vi "cmd check.vi"(8 "error in (no error)":errorcluster, 11 "motor in":refnum<class "AISAS motor.lvclass">) -> (0 "error out":errorcluster, 1 "Motor Ok?":bool, 3 "motor out":refnum<class "AISAS motor.lvclass">)   [LabVIEW 2014, in "AISAS motor.lvclass"]
uses:
  AISAS motor.lvclass
  Controls/motor.ctl
  AISAS motor.lvclass/AISAS motor.ctl
panel:
  out "Motor":T1
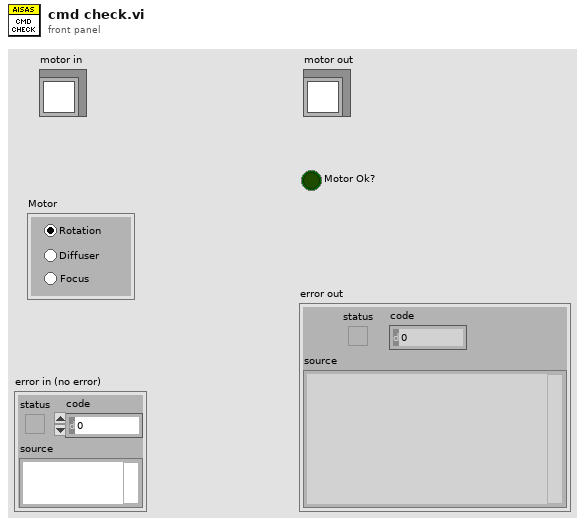
[diagram p1: front panel]
types:
  T1 = typedef "motor.ctl" = enum32{"Rotation", "Diffuser ", "Focus"}
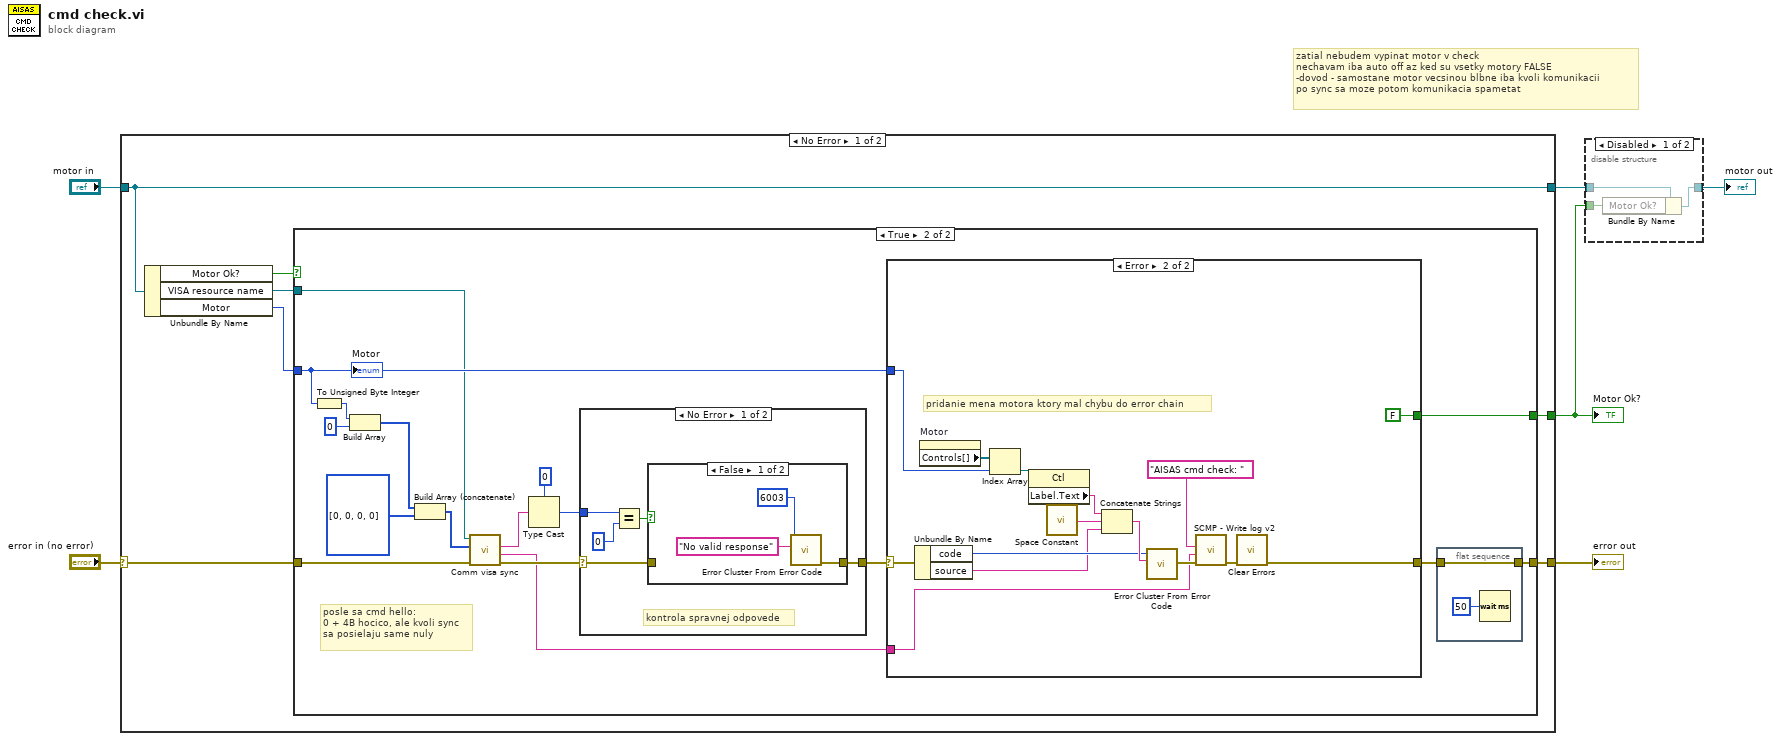
[diagram p0: block diagram]
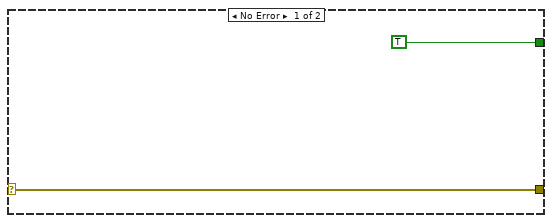
[diagram p4: hidden frame]
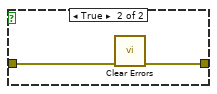
[diagram p5: hidden frame]
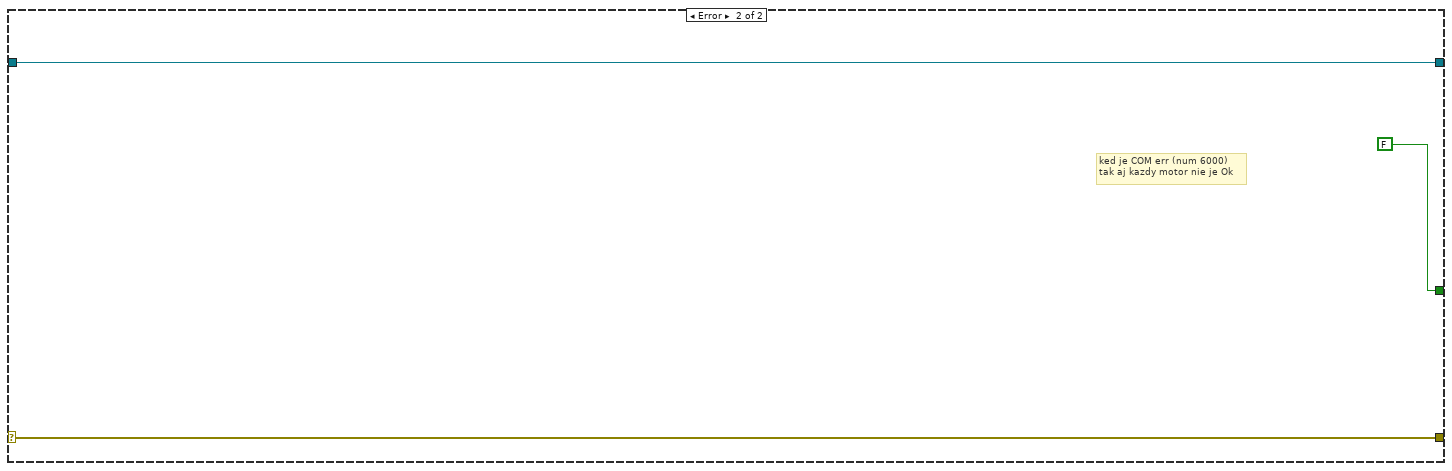
[diagram p7: hidden frame]
diagram:
  # "zatial nebudem vypinat motor v check\nnechavam iba auto off az ked su vsetky motory FALSE\n-dovod - samostane motor vecsinou blbne iba kvoli komunikacii\npo sync sa moze potom komunikacia spametat"
  n1 = case shown="No Error" "error in (no error)" {
    selector: "error in (no error)" -> [w11 w65]
    tunnel: [w13 w65] -> w5
    tunnel: "motor in" -> [w9 w64]
    tunnel: [w10 FALSE ("Motor Ok")] -> w3
    tunnel: [w9 w64] -> w2
    frame No Error {
      n2 = Unbundle By Name(w9) -> ("Motor Ok?"=w7:bool, "VISA resource name"=w8:refnum<visa-resource-name>, "Motor"=w12:T1)
      n3 = case shown="True" w7 {
        selector: w7 -> [w14 _]
        tunnel: [w14 w31] -> w10
        tunnel: [w15 w22] -> w13
        tunnel: w12 -> [_ w27]
        tunnel: w11 -> [w15 w25]
        tunnel: w8 -> [_ w16]
        frame False {
        }
        frame True {
          # "posle sa cmd hello:\n0 + 4B hocico, ale kvoli sync\nsa posielaju same nuly"
          n4 = To Unsigned Byte Integer(number=w27) -> (unsigned 8bit integer=w20:u8)
          n5 = Build Array(w20, u8 0) -> (w18:u8[])
          n6 = Build Array (concatenate)(w18, u8[] [0, 0, 0, 0]) -> (w17:u8[])
          n7 = call "Comm visa sync.vi"("error in (no error)"=w25, "Command"=w17, "VISA in"=w16) -> ("error out"=w30:errorcluster, "sync info"=w21:string, "Response"=w26:string)  [unwired: 5 in, 1 out]
          n8 = Type Cast(type=u8 0, x=w26) -> (*(type *) &x=w28:u8)
          n9 = case shown="No Error" w30 {
            selector: w30 -> [w56 w62]
            tunnel: [w54 w62] -> w32
            tunnel: w28 -> [w52 _]
            frame No Error {
              # "kontrola spravnej odpovede"
              n10 = Equal?(x=w52, y=u8 0) -> (x = y?=w55:bool)
              n11 = case shown="False" w55 {
                tunnel: w56 -> [_ w61]
                tunnel: [w57 w60] -> w54
                frame False {
                  n12 = call <vilib>:"Error Cluster From Error Code.vi"("error message (\"\")"="No valid response" ("error message (\"\")"), "error code (0)"=6003) -> ("error out"=w57:errorcluster)  [unwired: 7 in]
                }
                frame True {
                  n13 = call <vilib>:"Clear Errors.vi"("error in (no error)"=w61) -> ("error out"=w60:errorcluster)  [unwired: 5 in, 1 out]
                }
              }
            }
            frame Error {
            }
          }
          n14 = case shown="Error" w32 {
            selector: w32 -> [w35 w47]
            tunnel: [TRUE ("Motor Ok") FALSE ("Motor Ok")] -> w31
            tunnel: w27 -> [_ w48]
            tunnel: [w35 w37] -> w23
            tunnel: w21 -> [_ w38]
            frame No Error {
            }
            frame Error {
              # "pridanie mena motora ktory mal chybu do error chain"
              n15 = Unbundle By Name(w47) -> ("code"=w45:i32, "source"=w44:string)
              n16 = property on="Motor" class="RadioBtnsControl (strict)"() -> ("Controls[]"=w50:refnum<vi>[])  [unwired: 2 in, 2 out]
              n17 = Index Array(array=w50, index=w48) -> (element=w49:refnum<vi>)
              n18 = property class="Ctl"(reference=w49) -> ("Label.Text"=w43:string)  [unwired: 1 in, 2 out]
              n19 = call <vilib>:"Space Constant.vi"() -> ("String"=w42:string)
              n20 = Concatenate Strings(w43, w42, w44) -> (w46:string)
              n21 = call <vilib>:"Error Cluster From Error Code.vi"("error message (\"\")"=w46, "error code (0)"=w45) -> ("error out"=w41:errorcluster)  [unwired: 7 in]
              n22 = call "SCMP - Write log v2.vi"("Error to log"=w41, "data to end"=w38, "data"="AISAS cmd check: ") -> ("error out"=w39:errorcluster)  [unwired: 6 in, 2 out]
              n23 = call <vilib>:"Clear Errors.vi"("error in (no error)"=w39) -> ("error out"=w37:errorcluster)  [unwired: 5 in, 1 out]
            }
          }
          n24 = flat-sequence {
            tunnel: w23 -> [w34]
            tunnel: [w34] -> w22
            frame #0 {
              n25 = Wait (ms)(milliseconds to wait=u32 50) -> ()  [unwired: 1 out]
            }
          }
          "Motor" <- w27
        }
      }
    }
    frame Error {
      # "ked je COM err (num 6000)\ntak aj kazdy motor nie je Ok"
    }
  }
  "error out" <- w5
  "Motor Ok?" <- w3
  n26 = disable-structure shown="Disabled" {
    disable-tunnel: w3 -> [w68 _]
    disable-tunnel: w2 -> [w67 w69]
    disable-tunnel: [w66 w69] -> w1
    frame Disabled {
      n27 = Bundle By Name(cluster=w67, "Motor Ok?"=w68) -> (w66:refnum<class "AISAS motor.lvclass">)
    }
    frame Enabled {
    }
  }
  "motor out" <- w1
